vi "Write IP Address.vi"(10 "IP Address":string, 11 "Assert Service in":refnum<class "Assert Service.lvclass">) -> (3 "Assert Service out":refnum<class "Assert Service.lvclass">)   [LabVIEW 2016, in "Assert Service.lvlib" / "Assert Service.lvclass"]
uses:
  Assert Service.lvclass
  Assert Service.lvclass/Assert Service.ctl
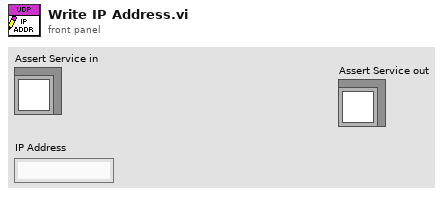
[diagram p1: front panel]
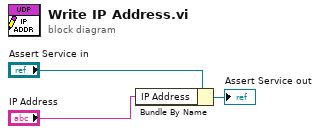
[diagram p0: block diagram]
diagram:
  n1 = Bundle By Name(cluster="Assert Service in", "IP Address"="IP Address") -> (→"Assert Service out":refnum<class "Assert Service.lvclass">)
